vi "Spex ScanMove.vi"(8 "error in":errorcluster, 9 "Moving Ref":refnum<vi>, 10 "Lambda Ref":refnum<vi>, 11 "Port":refnum<visa-resource-name>) -> (0 "error out":errorcluster, 1 "Wlenght":dbl caption="Wavelenght (nm)", 2 "SpexOut":string caption="Spex Output", 3 "VISA Resource Out":refnum<visa-resource-name>, 4 "Scan End":bool)   [LabVIEW 2010]
uses:
  <vilib>/Instr/_visa.llb/VISA Configure Serial Port (Instr).vi
  <userlib>/GenProg/WritebyWeakRefBool.vi
  <userlib>/GenProg/WritebyWeakRefNum.vi
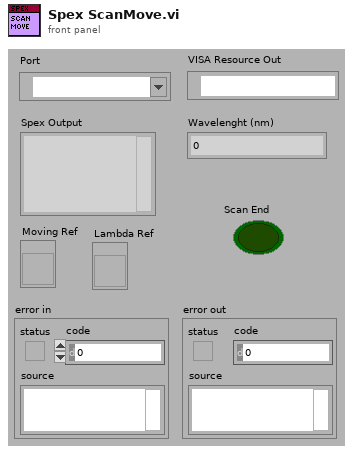
[diagram p1: front panel]
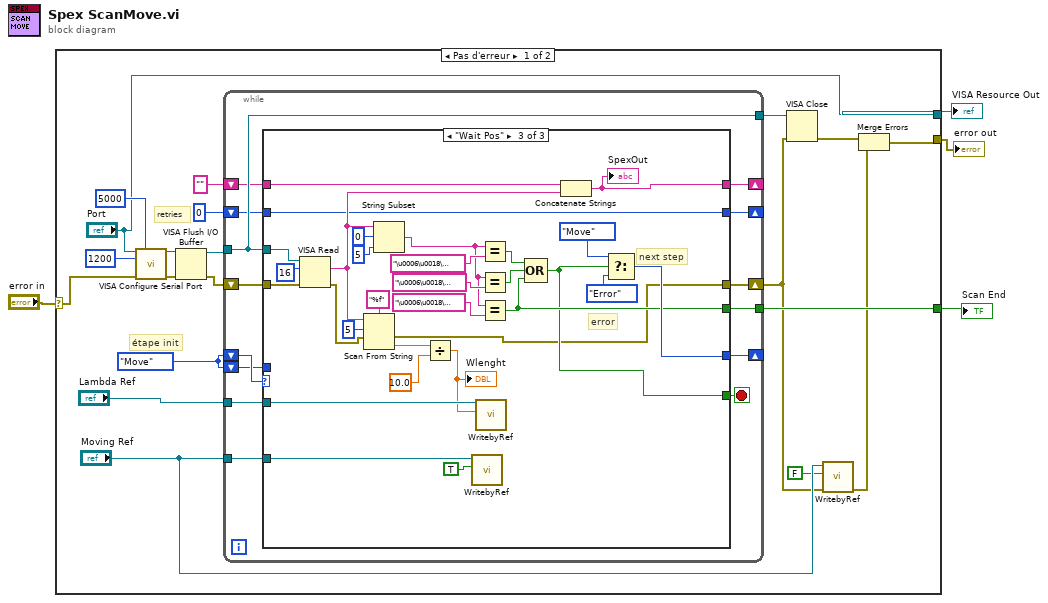
[diagram p0: block diagram]
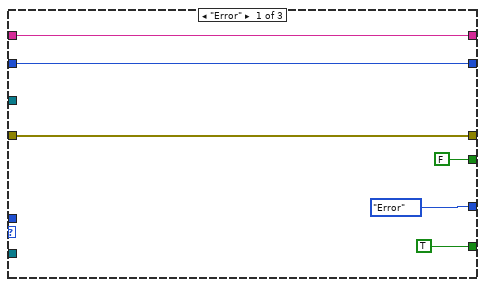
[diagram p2: hidden frame]
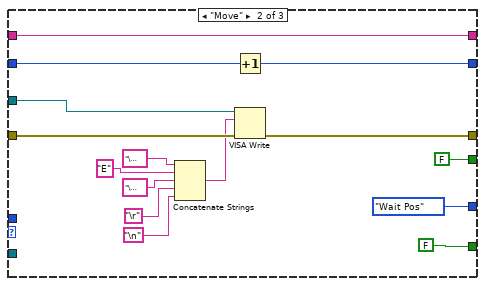
[diagram p3: hidden frame]
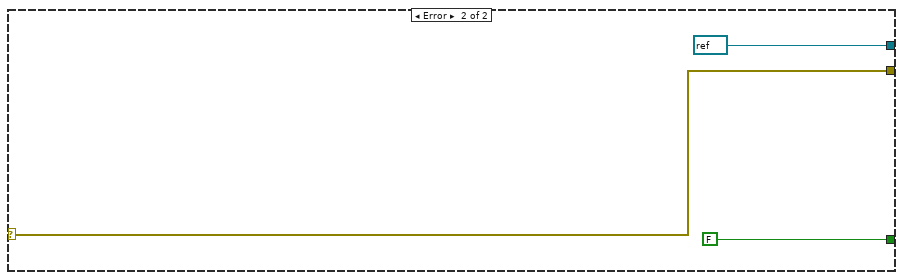
[diagram p4: hidden frame]
diagram:
  n1 = case shown="Pas d'erreur" "error in" {
    selector: "error in" -> [w16 w91]
    tunnel: [w6 w91] -> w1
    tunnel: ["Port" refnum<visa-resource-name> refnum ("VISA resource name out")] -> w3
    tunnel: [w21 FALSE] -> w2
    frame No Error {
      w23 = enum16{"Move", "Wait Pos", "Error"}."Move"
      # "retries"
      # "étape init"
      n2 = call-poly "VISA Configure Serial Port"("VISA resource name"="Port", "timeout (10sec)"=u32 5000, "baud rate (9600)"=u32 1200, "error in (no error)"=w16) -> ("VISA resource name out"=w18:refnum<visa-resource-name>, "error out"=w15:errorcluster)  [unwired: 10 in]
      n3 = VISA Flush I/O Buffer(VISA resource name=w18, error in (no error)=w15) -> (VISA resource name out=w17:refnum<visa-resource-name>, error out=w14:errorcluster)  [unwired: 1 in]
      n4 = while {
        shift-right: [w30] -> _
        shift-left: w23 -> [w38]
        tunnel: w17 -> [w34]
        shift-right: [w36] -> w7
        shift-left: w14 -> [w37]
        tunnel: [w34] -> w12
        shift-right: [w32] -> _
        shift-left: 0 -> [w33]
        shift-left: w23 -> [w31]
        shift-right: [w28] -> _
        shift-left: "" -> [w29]
        tunnel: [w27] -> w21
        tunnel: "Lambda Ref" -> [w26]
        tunnel: "Moving Ref" -> [w25]
        stop <- w35 stop-if-true
        n5 = case shown="\"Wait Pos\"" w38 {
          tunnel: w34 -> [_ w59 w89]
          tunnel: w37 -> [w41 w58 w88]
          tunnel: [w41 w57 w60] -> w36
          tunnel: [enum16{"Move", "Wait Pos", "Error"}."Error" enum16{"Move", "Wait Pos", "Error"}."Wait Pos" w77] -> w30
          tunnel: [TRUE FALSE w65] -> w35
          tunnel: w33 -> [w43 w55 w76]
          tunnel: [w43 w54 w76] -> w32
          tunnel: w31 -> [_ _ _]
          tunnel: w29 -> [w42 w53 w81]
          tunnel: [w42 w53 w79] -> w28
          tunnel: [FALSE FALSE w70] -> w27
          tunnel: w26 -> [_ _ w64]
          tunnel: w25 -> [_ _ w62]
          frame "Error" {
          }
          frame "Move" {
            n6 = Concatenate Strings("\u0018" ("string"), "E" ("string"), "\u0003" ("string"), "\r", "\n") -> (w45:string)
            n7 = Increment(x=w55) -> (x+1=w54:i32)
            n8 = VISA Write(VISA resource name=w59, write buffer=w45, error in (no error)=w58) -> (error out=w57:errorcluster)  [unwired: 2 out]
          }
          frame "Wait Pos" {
            # "error"
            # "next step"
            n9 = VISA Read(VISA resource name=w89, byte count=u32 16, error in (no error)=w88) -> (read buffer=w80:string, error out=w75:errorcluster)  [unwired: 2 out]
            n10 = Scan From String(format string="%f", input string=w80, initial scan location=u32 5, error in=w75) -> (error out=w60:errorcluster, output 1=w82:dbl)  [unwired: 1 in, 2 out]
            n11 = String Subset(string=w80, offset (0)=0, length (rest)=5 ("length (rest)")) -> (substring=w66:string)
            n12 = Divide(x=w82, y=10.0) -> (x/y=w63:dbl)
            "Wlenght" <- w63
            n13 = call-poly <userlib>:"WritebyRef.vi"("Valeur"=TRUE, "Control Ref"=w62) -> ()  [unwired: 9 in, 1 out]
            n14 = call-poly <userlib>:"WritebyRef.vi"("Valeur"=w63, "Control Ref"=w64) -> ()  [unwired: 9 in, 1 out]
            n15 = Equal?(x=w66, y="\u0006\u0018\u0002CA" ("x")) -> (x = y?=w78:bool)
            n16 = Equal?(x=w66, y="\u0006\u0018\u0002BA" ("x")) -> (x = y?=w74:bool)
            n17 = Equal?(x=w66, y="\u0006\u0018\u0002EA" ("x")) -> (x = y?=w70:bool)
            n18 = Compound Arithmetic op=OR(w78, w74, w70) -> (w65:bool)
            n19 = Concatenate Strings(w81, w80) -> (w79:string)
            "SpexOut" <- w79
            n20 = Select(t=enum16{"Move", "Wait Pos", "Error"}."Move", s=w65, f=enum16{"Move", "Wait Pos", "Error"}."Error") -> (s? t:f=w77:enum16{"Move", "Wait Pos", "Error"})
          }
        }
      }
      n21 = VISA Close(VISA resource name=w12, error in (no error)=w7) -> (error out=w13:errorcluster)
      n22 = call-poly <userlib>:"WritebyRef.vi"("error in"=w7, "Valeur"=FALSE, "Control Ref"="Moving Ref") -> ("error out"=w5:errorcluster)  [unwired: 8 in]
      n23 = Merge Errors(w13, w5) -> (w6:errorcluster)
    }
    frame Error {
    }
  }
  "error out" <- w1
  "VISA Resource Out" <- w3
  "Scan End" <- w2
